vi "Read Private Thread Error.vi"(8 "error in (no error)":errorcluster, 10 "private thread index":i32, 11 "Thread Manager in":refnum<class "Thread Manager.lvclass">) -> (0 "error out":errorcluster, 2 "thread error":errorcluster, 3 "Thread Manager out":refnum<class "Thread Manager.lvclass">)   [LabVIEW 2019, in "DSF Core.lvlib" / "Thread Manager.lvclass"]
uses:
  Thread Manager.lvclass
  Thread Manager.lvclass/Thread Manager.ctl
  Thread/Thread.lvclass
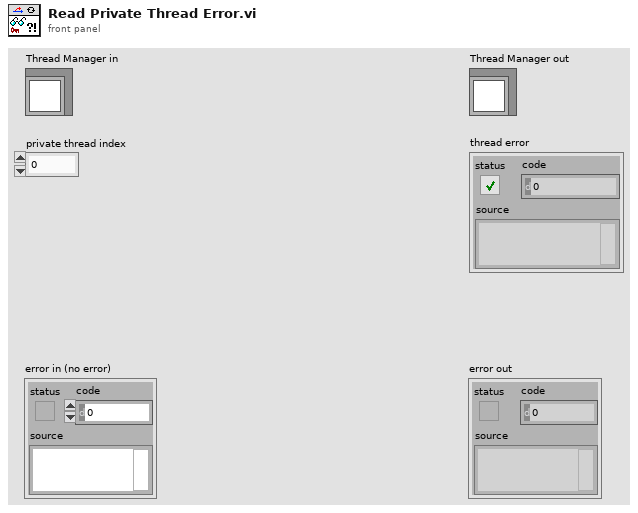
[diagram p1: front panel]
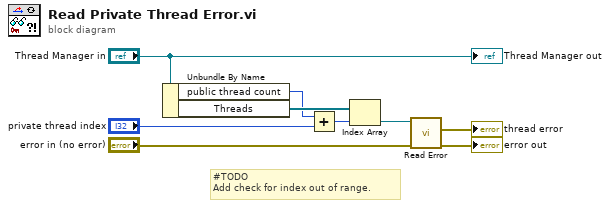
[diagram p0: block diagram]
diagram:
  # "#TODO\nAdd check for index out of range."
  n1 = Unbundle By Name("Thread Manager in") -> ("public thread count"=w1:i32, "Threads"=w4:refnum<class "Thread.lvclass">[])
  n2 = Add(x=w1, y="private thread index") -> (x+y=w2:i32)
  n3 = Index Array(array=w4, index=w2) -> (element=w8:refnum<class "Thread.lvclass">)
  n4 = call "Read Error.vi"("error in (no error)"="error in (no error)", "Thread in"=w8) -> ("error out"=→"error out":errorcluster, "error"=→"thread error":errorcluster)  [unwired: 7 in, 1 out]
  "Thread Manager out" <- "Thread Manager in"
